vi "NonUtilisedTime.vi"(0 "Event Name":string, 5 "Previous Event Time":string, 7 "Event Time":string, 9 "Previous Event Name":string) -> (4 "Non Utilized Time":string)   [LabVIEW 2019, in "DataLogger.lvclass"]
uses:
  DataLogger.lvclass
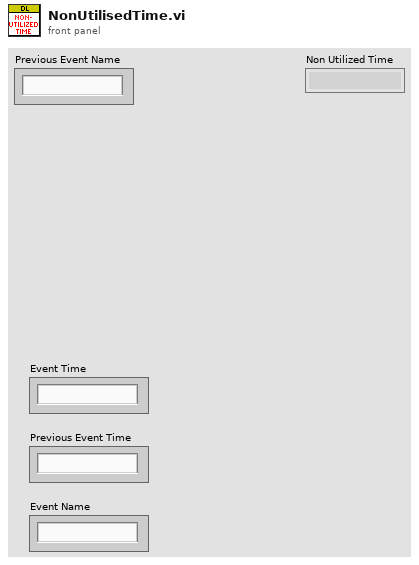
[diagram p1: front panel]
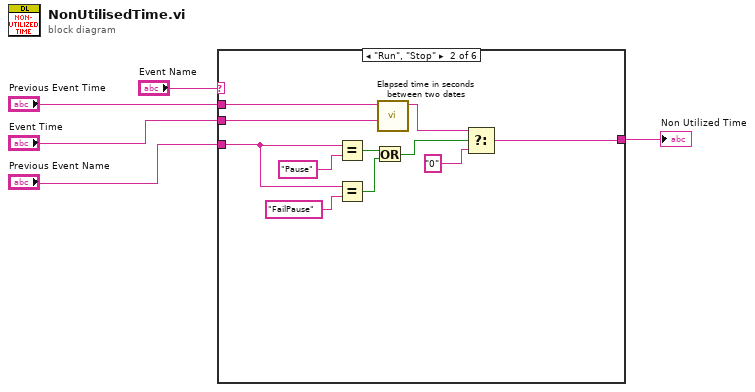
[diagram p0: block diagram]
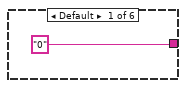
[diagram p2: hidden frame]
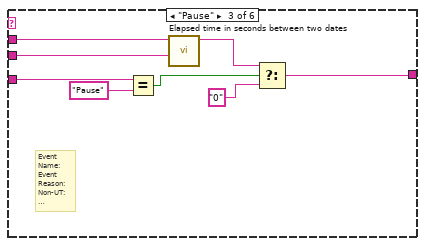
[diagram p3: hidden frame]
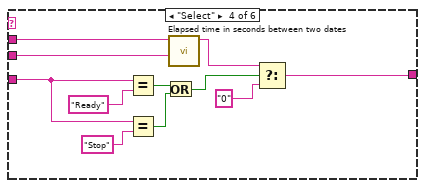
[diagram p4: hidden frame]
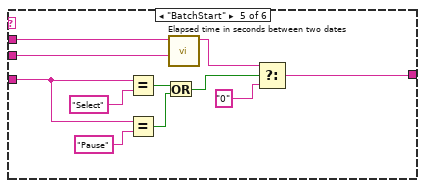
[diagram p5: hidden frame]
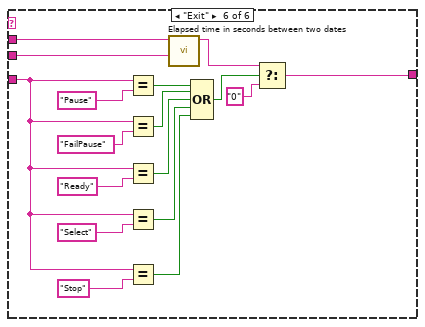
[diagram p6: hidden frame]
diagram:
  n1 = case shown="\"Run\", \"Stop\"" "Event Name" {
    tunnel: "Previous Event Name" -> [_ w11 w20 w30 w41 w54]
    tunnel: ["0" w17 w25 w36 w47 w64] -> w1
    tunnel: "Previous Event Time" -> [_ w14 w22 w33 w44 w61]
    tunnel: "Event Time" -> [_ w13 w21 w32 w43 w60]
    frame Default {
    }
    frame "Run", "Stop" {
      n2 = Equal?(x=w11, y="Pause") -> (x = y?=w8:bool)
      n3 = Equal?(x=w11, y="FailPause") -> (x = y?=w9:bool)
      n4 = Or(x=w8, y=w9) -> (x .or. y?=w7:bool)
      n5 = call "Elapsed time in seconds between two dates.vi"("Start Date/Time"=w14, "End Date/Time"=w13) -> ("Time difference in Seconds"=w15:string)  [unwired: 8 in]
      n6 = Select(t=w15, s=w7, f="0") -> (s? t:f=w17:string)
    }
    frame "Pause" {
      # "Event Name:       Event Reason:                                                                   Non-UT:\n\n1 .Pause                   Lunch Break                                                                         0\n\n2. Pause                   Accidental Press                                                                Some N.U.T(From Pause to pause)\n                                 (On cancel button press on Stop PopUp) \n\n3. Run                       Accidental Press                                                                 From Pause to Run"
      n7 = Equal?(x=w20, y="Pause") -> (x = y?=w18:bool)
      n8 = call "Elapsed time in seconds between two dates.vi"("Start Date/Time"=w22, "End Date/Time"=w21) -> ("Time difference in Seconds"=w23:string)  [unwired: 8 in]
      n9 = Select(t=w23, s=w18, f="0") -> (s? t:f=w25:string)
    }
    frame "Select" {
      n10 = Equal?(x=w30, y="Ready") -> (x = y?=w27:bool)
      n11 = Equal?(x=w30, y="Stop") -> (x = y?=w28:bool)
      n12 = Or(x=w27, y=w28) -> (x .or. y?=w26:bool)
      n13 = call "Elapsed time in seconds between two dates.vi"("Start Date/Time"=w33, "End Date/Time"=w32) -> ("Time difference in Seconds"=w34:string)  [unwired: 8 in]
      n14 = Select(t=w34, s=w26, f="0") -> (s? t:f=w36:string)
    }
    frame "BatchStart" {
      n15 = Equal?(x=w41, y="Select") -> (x = y?=w38:bool)
      n16 = Equal?(x=w41, y="Pause") -> (x = y?=w39:bool)
      n17 = Or(x=w38, y=w39) -> (x .or. y?=w37:bool)
      n18 = call "Elapsed time in seconds between two dates.vi"("Start Date/Time"=w44, "End Date/Time"=w43) -> ("Time difference in Seconds"=w45:string)  [unwired: 8 in]
      n19 = Select(t=w45, s=w37, f="0") -> (s? t:f=w47:string)
    }
    frame "Exit" {
      n20 = Equal?(x=w54, y="Pause") -> (x = y?=w52:bool)
      n21 = Equal?(x=w54, y="FailPause") -> (x = y?=w51:bool)
      n22 = Equal?(x=w54, y="Ready") -> (x = y?=w50:bool)
      n23 = Equal?(x=w54, y="Select") -> (x = y?=w49:bool)
      n24 = Equal?(x=w54, y="Stop") -> (x = y?=w48:bool)
      n25 = call "Elapsed time in seconds between two dates.vi"("Start Date/Time"=w61, "End Date/Time"=w60) -> ("Time difference in Seconds"=w62:string)  [unwired: 8 in]
      n26 = Compound Arithmetic op=OR(w52, w51, w50, w49, w48) -> (w53:bool)
      n27 = Select(t=w62, s=w53, f="0") -> (s? t:f=w64:string)
    }
  }
  "Non Utilized Time" <- w1
